vi "check NVH error.vi"(8 "Error Table In":string[][](table)=[["", "", ""]]) -> (0 "NVH Error?":bool, 2 "have errror?":bool)   [LabVIEW 2018]
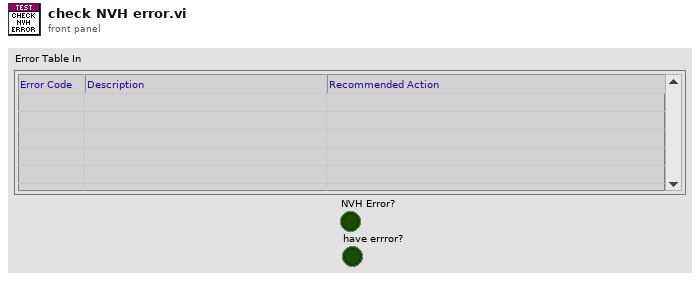
[diagram p1: front panel]
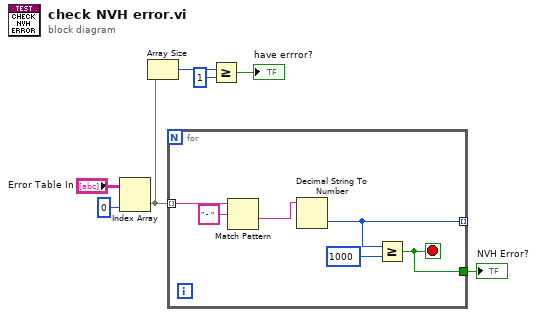
[diagram p0: block diagram]
diagram:
  n1 = Index Array(array="Error Table In", index (col)=0 ("disabled index (col)")) -> (element=w2:string[])  [unwired: 1 in]
  n2 = Array Size(array=w2) -> (size(s)=w4:i32)
  n3 = for {
    tunnel: w2 -> [w13] mode=indexing
    tunnel: [w10] -> _ mode=indexing
    tunnel: [w8] -> w6
    stop <- w8 stop-if-true
    n4 = Match Pattern(string=w13, regular expression=" - ") -> (after substring=w11:string)  [unwired: 1 in, 3 out]
    n5 = Decimal String To Number(string=w11) -> (number=w10:i32)  [unwired: 2 in, 1 out]
    n6 = Greater Or Equal?(x=w10, y=1000) -> (x >= y?=w8:bool)
  }
  "NVH Error?" <- w6
  n7 = Greater Or Equal?(x=w4, y=1 ("disabled index (col)")) -> (x >= y?=→"have errror?":bool)
